vi "V-Meter Measure (3706).vi"(7 "Slot Number":u8=1 min=1 max=6, 8 "error in (no error)":errorcluster, 10 "Boolean":bool, 11 "VISA resource name in":refnum<visa-resource-name>) -> (0 "error out":errorcluster, 2 "Measurement":dbl, 3 "VISA resource name out":refnum<visa-resource-name>)   [LabVIEW 2016, in "Hall Effect Library.lvlib"]
uses:
  Hall Effect Library.lvlib
  Global Variables/Test Settings.vi
  <instrlib>/Keithley 3706/Keithley 3706.lvlib
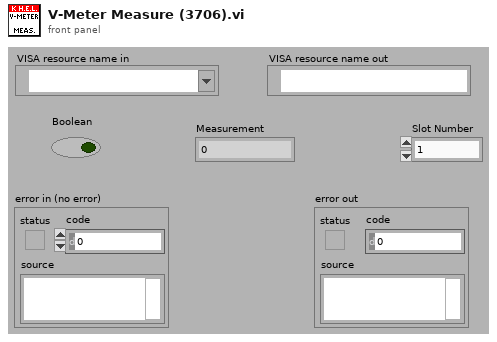
[diagram p1: front panel]
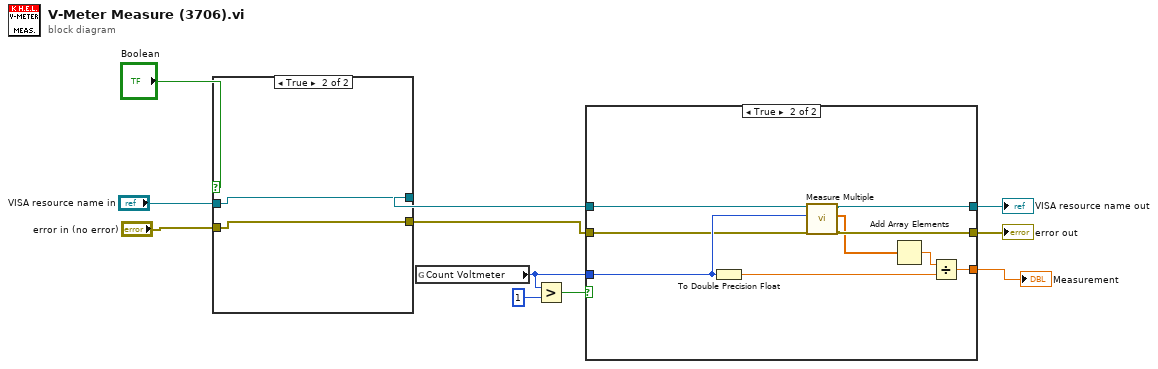
[diagram p0: block diagram]
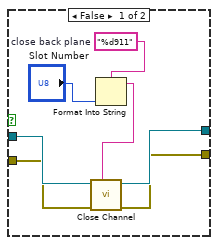
[diagram p2: hidden frame]
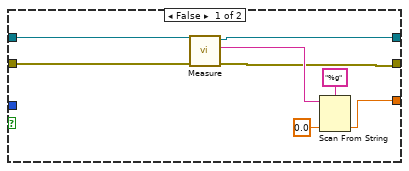
[diagram p3: hidden frame]
diagram:
  n1 = case shown="True" "Boolean" {
    tunnel: "VISA resource name in" -> [w18 w20]
    tunnel: "error in (no error)" -> [w17 w19]
    tunnel: [w16 w20] -> w2
    tunnel: [w15 w19] -> w1
    frame False {
      w14 = "%d911"  # close back plane
      n2 = Format Into String(format string=w14, "Slot Number") -> (resulting string=w12:string)  [unwired: 2 in, 1 out]
      n3 = call <instrlib>:"Close Channel.vi"("Channel List"=w12, "error in (no error)"=w17, "VISA resource name"=w18) -> ("error out"=w15:errorcluster, "VISA resource name out"=w16:refnum<visa-resource-name>)  [unwired: 7 in]
    }
    frame True {
    }
  }
  n4 = global read "Test Settings.vi" "Count Voltmeter"() -> (w7:i32)
  n5 = Greater?(x=w7, y=1) -> (0:w10:bool)
  n6 = case shown="True" w10 {
    tunnel: w1 -> [w21 w29]
    tunnel: w2 -> [w22 w30]
    tunnel: [w23 w32] -> w9
    tunnel: [w24 w33] -> w8
    tunnel: w7 -> [_ w34]
    tunnel: [w26 w35] -> w6
    frame False {
      n7 = call <instrlib>:"Measure.vi"("error in (no error)"=w21, "VISA resource name"=w22) -> ("error out"=w24:errorcluster, "Output"=w25:string, "VISA resource name out"=w23:refnum<visa-resource-name>)  [unwired: 7 in]
      n8 = Scan From String(format string="%g", input string=w25, default 1=0.0 ("default value 1")) -> (output 1=w26:dbl)  [unwired: 2 in, 3 out]
    }
    frame True {
      n9 = To Double Precision Float(number=w34) -> (double precision float=w36:dbl)
      n10 = call <instrlib>:"Measure Multiple.vi"("error in (no error)"=w29, "Measure Count"=w34, "VISA resource name"=w30) -> ("error out"=w33:errorcluster, "Data"=w31:dbl[], "VISA resource name out"=w32:refnum<visa-resource-name>)  [unwired: 6 in]
      n11 = Add Array Elements(numeric array=w31) -> (sum=w37:dbl)
      n12 = Divide(x=w37, y=w36) -> (x/y=w35:dbl)
    }
  }
  "error out" <- w8
  "VISA resource name out" <- w9
  "Measurement" <- w6
